vi "Add Name-UserEvent.vi"(9 "UserEvent":T1, 10 "Name":string, 11 "UserEventTimer in":refnum<class "TimerEngine.lvclass">) -> (3 "UserEventTimer out":refnum<class "TimerEngine.lvclass">)   [LabVIEW 2017, in "TimerEngine.lvlib" / "TimerEngine.lvclass"]
uses:
  TimerEngine.lvclass
  _Typedef/Timer-UserEvent.ctl
  TimerEngine.lvclass/TimerEngine.ctl
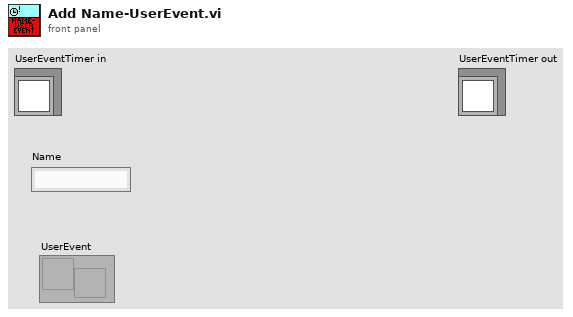
[diagram p1: front panel]
types:
  T1 = typedef "TimerEngine.lvlib/TimerEngine.lvclass/Timer-Userevent.ctl" = refnum<user-event>
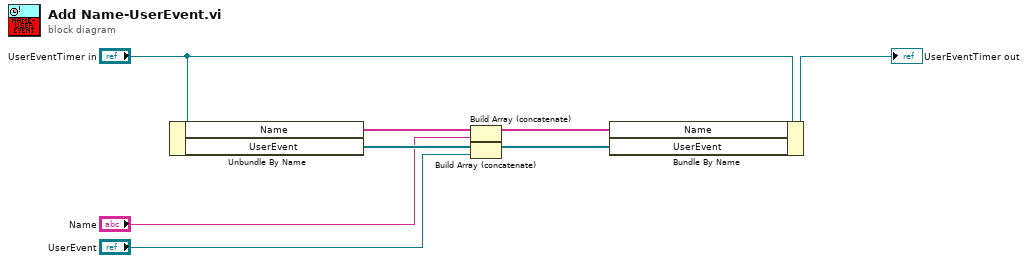
[diagram p0: block diagram]
diagram:
  n1 = Unbundle By Name("UserEventTimer in") -> ("Name"=w6:string[], "UserEvent"=w5:T1[])
  n2 = Build Array (concatenate)(w6, "Name") -> (w4:string[])
  n3 = Build Array (concatenate)(w5, "UserEvent") -> (w3:T1[])
  n4 = Bundle By Name(cluster="UserEventTimer in", "Name"=w4, "UserEvent"=w3) -> (→"UserEventTimer out":refnum<class "TimerEngine.lvclass">)
